vi "AscIIToChar(Byte Array to String).vi"(1 "ASCII":u8 format="DEC:%2d\nHEX:%2x") -> (0 "Char":string)   [LabVIEW 2012]
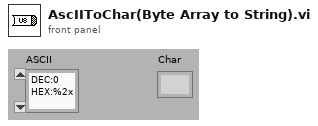
[diagram p1: front panel]
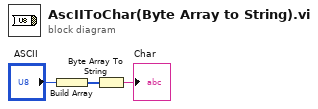
[diagram p0: block diagram]
diagram:
  n1 = Build Array("ASCII") -> (w2:u8[])
  n2 = Byte Array To String(unsigned byte array=w2) -> (string=→"Char":string)
